vi "dsc9513SetLoadRegister.vi"(8 "error in":errorcluster, 9 "value":u16, 10 "counter":u8=1 min=1 max=10, 11 "board":i16) -> (0 "error out":errorcluster, 3 "boardOut":i16)   [LabVIEW 2011, in "Diamond Universal Driver.lvlib"]
doc: "This function loads the supplied data into the specified counter's Load register. The Load register is used to specify a counter's initial value as well as to set the reload value when the counter reaches its terminal count during repetitive counting modes. The data is not actually loaded into the counter's count register until a Load or Load and Arm command is issued with dsc9513CounterControl()."
uses:
  Diamond Universal Driver.lvlib
  Controls/error codes.ctl
  Instruments/WL OPC/Support/dlls/dscud.dll
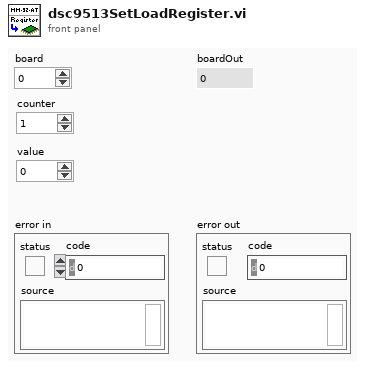
[diagram p1: front panel]
types:
  T1 = typedef "Diamond Universal Driver.lvlib/error codes.ctl" = enum8{"DE_NONE", "DE_HW_FAILURE", "DE_SW_FAILURE", "DE_HW_NOT_SUPPORTED", "DE_SW_NOT_SUPPORTED", "DE_INVALID_PARM", "DE_ALTERNATE_IN_PROGRESS", "DE_NONE_IN_PROGRESS", "DE_BUFFER_ROLLOVER", "DE_INVALID_ERROR_CODE", "DE_ALREADY_PAUSED", "DE_OVERFLOW", "DE_INVALID_FUNC", "DE_DSCUDH_INVALID", "DE_INVALID_BOARD", "DE_BOARD_LIMIT_REACHED", "DE_BOARD_BUSY", "DE_INVALID_WINDRVR_HANDLE", "DE_INVALID_WINDRVR_VERSION", "DE_BAD_WINDRVR_BOARD_INIT", "DE_OPERATION_TIMED_OUT", "DE_INVALID_WINDRVR_KP", "DE_THREAD_FAILURE"}
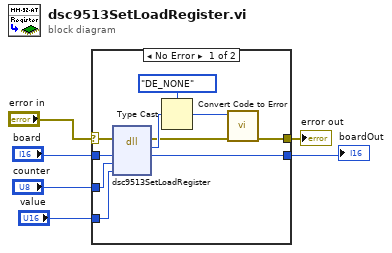
[diagram p0: block diagram]
diagram:
  n1 = case shown="No Error" "error in" {
    selector: "error in" -> [w13 w18]
    tunnel: "board" -> [w11 w17]
    tunnel: [w10 w17] -> w4
    tunnel: [w9 w18] -> w3
    tunnel: "value" -> [w8 _]
    tunnel: "counter" -> [w7 _]
    frame No Error {
      n2 = dll-call lib="C:/Users/mrichardson/Documents/Web Based Version Control SW/Instruments/WL OPC/Support/dlls/dscud.dll" fn="dsc9513SetLoadRegister"(error in=w13, "board"=w11, "counter"=w7, "value"=w8) -> (error out=w12:errorcluster, "error"=w14:u8, "board"=w10:i16)  [unwired: 4 in, 1 out]
      n3 = Type Cast(type=error_codes."DE_NONE" ("error codes"), x=w14) -> (*(type *) &x=w16:T1)
      n4 = call "Convert Code to Error.vi"("error in"=w12, "error codes"=w16) -> ("error out"=w9:errorcluster)  [unwired: 9 in]
    }
    frame Error {
    }
  }
  "boardOut" <- w4
  "error out" <- w3
